vi "ABAPI Dist Create Directory Recursive.vi"(4 "error in (no error)":errorcluster, 5 "permissions (111101101)":i16=493 format="%b", 7 "directory":path) -> (0 "error out":errorcluster, 2 "Directories Created":path[](array[path]), 3 "directory copy":path)   [LabVIEW 2020]
uses:
  <resource>/Framework/Providers/Common/provcom_StringGlobals.vi
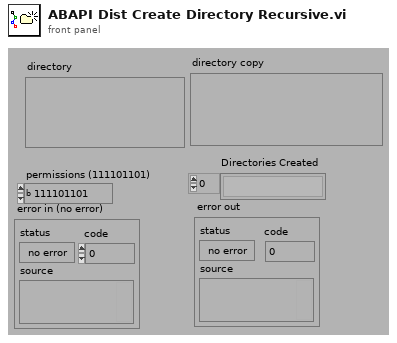
[diagram p1: front panel]
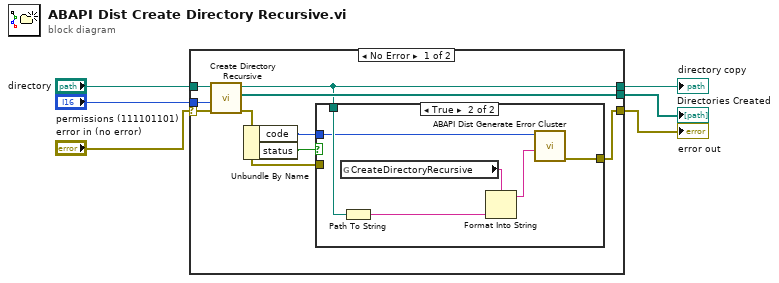
[diagram p0: block diagram]
diagram:
  n1 = case shown="No Error" "error in (no error)" {
    selector: "error in (no error)" -> [w12 w23]
    tunnel: "directory" -> [w15 w24]
    tunnel: "permissions (111101101)" -> [w14 _]
    tunnel: [w11 w24] -> w4
    tunnel: [w13 _] -> w3
    tunnel: [w8 w23] -> w2
    frame No Error {
      n2 = call <vilib>:"Create Directory Recursive.vi"("error in (no error)"=w12, "permissions"=w14, "directory"=w15) -> ("error out"=w7:errorcluster, "directories created"=w13:path[], "directory copy"=w11:path)  [unwired: 2 in]
      n3 = Unbundle By Name(w7) -> ("code"=w9:i32, "status"=w10:bool)
      n4 = case shown="True" w10 {
        tunnel: w11 -> [_ w22]
        tunnel: w9 -> [_ w20]
        tunnel: [w16 w17] -> w8
        tunnel: w7 -> [w16 _]
        frame False {
        }
        frame True {
          n5 = global read "provcom_StringGlobals.vi" "CreateDirectoryRecursive"() -> (w21:string)
          n6 = Path To String(path=w22) -> (string=w19:string)
          n7 = Format Into String(format string=w21, w19) -> (resulting string=w18:string)  [unwired: 2 in, 1 out]
          n8 = call <vilib>:"ABAPI Dist Generate Error Cluster.vi"("Additional Message"=w18, "Code"=w20) -> ("error out"=w17:errorcluster)  [unwired: 9 in]
        }
      }
    }
    frame Error {
    }
  }
  "directory copy" <- w4
  "error out" <- w2
  "Directories Created" <- w3
